vi "Single PWM.vi"() -> ()   [LabVIEW 2020, in "CTI-Scratchpad.lvlib"]
uses:
  CTI-Scratchpad.lvlib
  CTI/GPIO Number.ctl
  CTI/PWM/PWM.lvclass/PWM.ctl
  CTI/GPIO/GPIO.lvclass/GPIO.ctl
  CTI/PWM/GPIO Number.vi
  CTI/GPIO/GPIO Number.vi
  CTI/Session/PWM Write Frequency.vi
  CTI/Session/PWM Read Frequency.vi
  CTI/Session/Session.lvclass
  CTI/VisaComms/VisaComms.lvclass
  CTI/PWM/PWM.lvclass
  CTI/CTI.lvlib
panel:
  out "Act. Freq":sgl format="%.4f"
  out "Act. Duty":sgl format="%_6f"
  in  "Frequency":sgl(slide) scale=10.0..500000.0
  in  "stop":bool
  in  "Port":refnum<visa-resource-name>="COM3"
  in  "Duty":sgl(slide) scale=0.0..1.0
  in  "Channel":T1
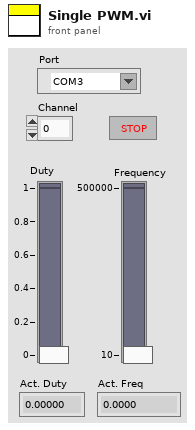
[diagram p1: front panel]
types:
  T1 = typedef "CTI.lvlib/GPIO Number.ctl" = i8
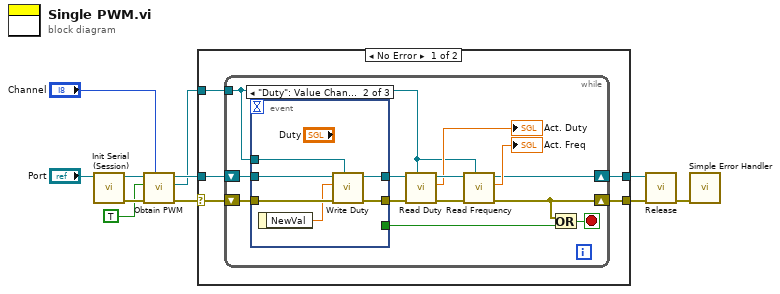
[diagram p0: block diagram]
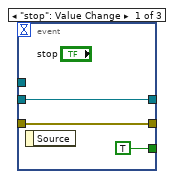
[diagram p2: hidden frame]
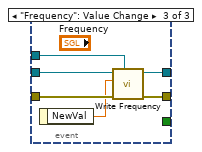
[diagram p3: hidden frame]
diagram:
  n1 = call "Init Serial (Session).vi"("VISA resource name in"="Port") -> ("error out"=w9:errorcluster, "Session"=w10:refnum<class "Session.lvclass">)  [unwired: 9 in]
  n2 = call "Obtain PWM.vi"("GPIO #"="Channel", "error in (no error)"=w9, "Enable (F)"=TRUE, "Session in"=w10) -> ("error out"=w8:errorcluster, "PWM"=w1:refnum<class "PWM.lvclass">, "Session out"=w7:refnum<class "Session.lvclass">)  [unwired: 5 in]
  n3 = case shown="No Error" w8 {
    selector: w8 -> [w15 w45]
    tunnel: w7 -> [w16 w46]
    tunnel: [w14 w46] -> w5
    tunnel: [w13 w45] -> w6
    tunnel: w1 -> [w12 _]
    frame No Error {
      n4 = while {
        shift-right: [w18] -> w14
        shift-left: w16 -> [w28]
        shift-right: [w19] -> w13
        shift-left: w15 -> [w27]
        tunnel: w12 -> [w17]
        stop <- w29 stop-if-true
        n5 = event shown="[1] \"Duty\": Value Change" {
          selector: _ -> [_ _ _]
          dyn-events: _ -> [_ _ _]
          timeout: _ -> [_ _ _]
          tunnel: [w32 w36 w42] -> w25
          tunnel: w28 -> [w32 w38 w44]
          tunnel: [w31 w35 w41] -> w23
          tunnel: w27 -> [w31 w37 w43]
          tunnel: [TRUE _ _] -> w26
          tunnel: w17 -> [_ w34 w40]
          event "stop": Value Change {
            n6 = event-data() -> ()  [unwired: 1 in, 1 out]
          }
          event "Duty": Value Change {
            n7 = event-data() -> ("NewVal"=w33:sgl)  [unwired: 1 in]
            n8 = call "Write Duty.vi"("PWM"=w34, "error in (no error)"=w37, "Duty % (0-1)"=w33, "Session In"=w38) -> ("error out"=w35:errorcluster, "Session Out"=w36:refnum<class "Session.lvclass">)  [unwired: 6 in]
          }
          event "Frequency": Value Change {
            n9 = event-data() -> ("NewVal"=w39:sgl)  [unwired: 1 in]
            n10 = call "Write Frequency.vi"("PWM"=w40, "error in (no error)"=w43, "Frequency Hz"=w39, "Session In"=w44) -> ("error out"=w41:errorcluster, "Session Out"=w42:refnum<class "Session.lvclass">)  [unwired: 6 in]
          }
        }
        n11 = call "Read Duty.vi"("PWM"=w17, "error in (no error)"=w23, "Session In"=w25) -> ("error out"=w20:errorcluster, "Duty % (0-1)"=→"Act. Duty":sgl, "Session Out"=w24:refnum<class "Session.lvclass">)  [unwired: 6 in]
        n12 = call "Read Frequency.vi"("PWM"=w17, "error in (no error)"=w20, "Session In"=w24) -> ("error out"=w19:errorcluster, "Frequency Hz"=→"Act. Freq":sgl, "Session Out"=w18:refnum<class "Session.lvclass">)  [unwired: 6 in]
        n13 = Or(x=w19, y=w26) -> (x .or. y?=w29:bool)
      }
    }
    frame Error {
    }
  }
  n14 = call-dynamic "Release.vi"("error in (no error)"=w6, "Session in"=w5) -> ("error out"=w4:errorcluster)  [unwired: 9 in]
  n15 = call <vilib>:"Simple Error Handler.vi"("error in (no error)"=w4) -> ()  [unwired: 4 in, 5 out]
